vi "Parse GSA Sentence.vi"(8 "error in (no error)":errorcluster, 11 "GSA sentence":string) -> (0 "error out":errorcluster, 3 "GSA data":T1 {"type of fix"."mode" items=["", "No Fix", "2D Fix", "3D Fix"]; "selection of fix"."selection of 2D or 3D fix" items=["Automatic", "Manual"]})   [LabVIEW 2011, in "u-blox 5 Series.lvlib"]
doc: "Returns data contained in an NMEA sentence. You must manually select the polymorphic instance to use."
uses:
  u-blox 5 Series.lvlib
  typedefs/GSA Data.ctl
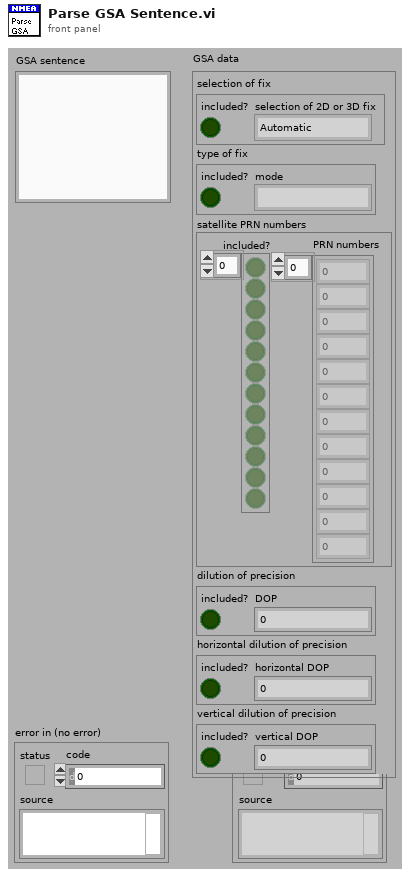
[diagram p1: front panel]
types:
  T1 = typedef "u-blox 5 Series.lvlib/GSA Data.ctl" = cluster{"selection of fix":cluster{"included?":bool, "selection of 2D or 3D fix":u16}, "type of fix":cluster{"included?":bool, "mode":u16}, "satellite PRN numbers":cluster{"included?":bool[], "PRN numbers":i32[]}, "dilution of precision":cluster{"included?":bool, "DOP":dbl}, "horizontal dilution of precision":cluster{"included?":bool, "horizontal DOP":dbl}, "vertical dilution of precision":cluster{"included?":bool, "vertical DOP":dbl}}
  T2 = cluster{"Included?":bool[], "Satellite PRNs":i32[]}
  T3 = cluster{"Valid?":bool, "Selection of 2D or 3D Fix":u16}
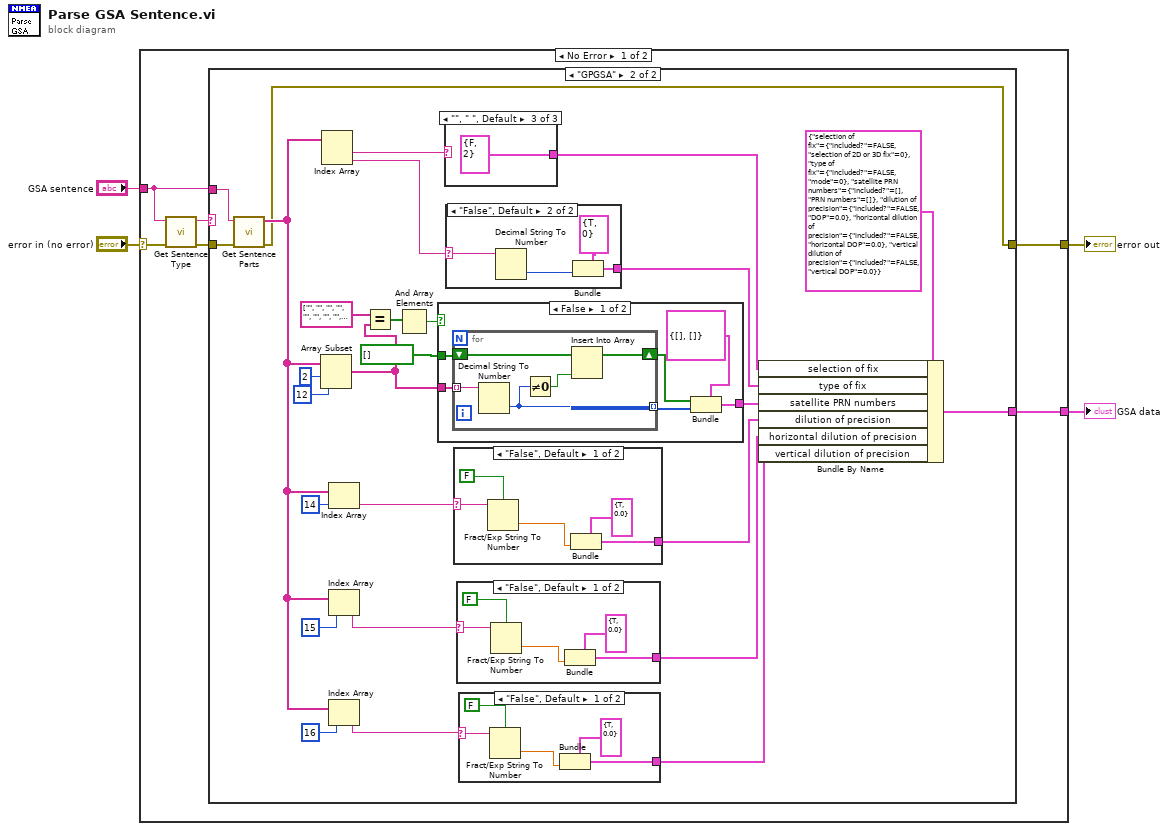
[diagram p0: block diagram]
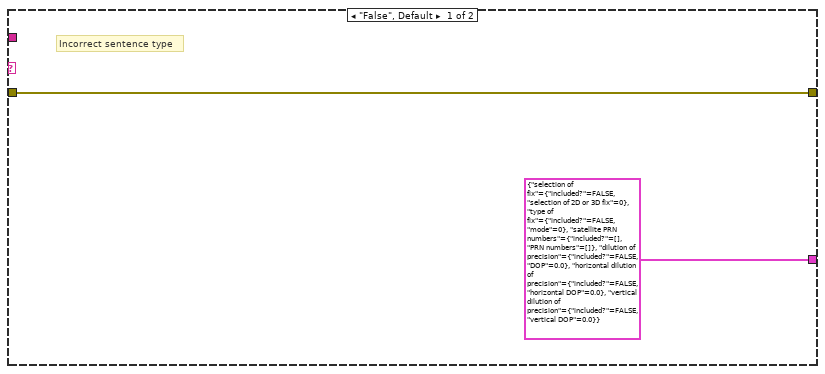
[diagram p2: hidden frame]
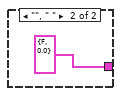
[diagram p3: hidden frame]
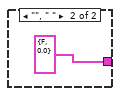
[diagram p4: hidden frame]
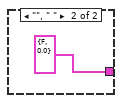
[diagram p5: hidden frame]
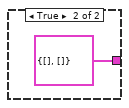
[diagram p6: hidden frame]
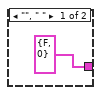
[diagram p7: hidden frame]
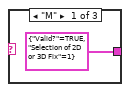
[diagram p8: hidden frame]
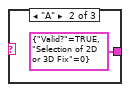
[diagram p9: hidden frame]
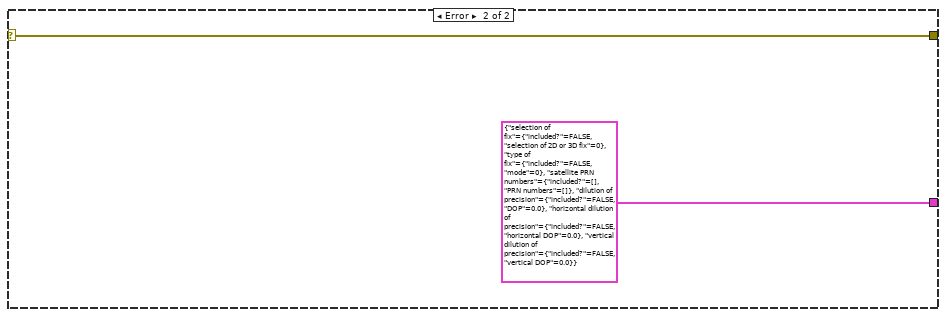
[diagram p10: hidden frame]
diagram:
  n1 = case shown="No Error" "error in (no error)" {
    selector: "error in (no error)" -> [w8 w79]
    tunnel: [w9 w79] -> w2
    tunnel: [w10 T1 {"selection of fix"={"included?"=FALSE, "selection of 2D or 3D fix"=0}, "type of fix"={"included?"=FALSE, "mode"=0}, "satellite PRN numbers"={"included?"=[], "PRN numbers"=[]}, "dilution of precision"={"included?"=FALSE, "DOP"=0.0}, "horizontal dilution of precision"={"included?"=FALSE, "horizontal DOP"=0.0}, "vertical dilution of precision"={"included?"=FALSE, "vertical DOP"=0.0}} ("GSA Data")] -> w1
    tunnel: "GSA sentence" -> [w6 _]
    frame No Error {
      n2 = call "Get Sentence Type.vi"("error in (no error)"=w8, "sentence"=w6) -> ("error out"=w7:errorcluster, "sentence type"=w5:string)  [unwired: 1 in, 7 out]
      n3 = case shown="\"GPGSA\"" w5 {
        tunnel: w6 -> [_ w14]
        tunnel: w7 -> [w11 w39]
        tunnel: [T1 {"selection of fix"={"included?"=FALSE, "selection of 2D or 3D fix"=0}, "type of fix"={"included?"=FALSE, "mode"=0}, "satellite PRN numbers"={"included?"=[], "PRN numbers"=[]}, "dilution of precision"={"included?"=FALSE, "DOP"=0.0}, "horizontal dilution of precision"={"included?"=FALSE, "horizontal DOP"=0.0}, "vertical dilution of precision"={"included?"=FALSE, "vertical DOP"=0.0}} ("GSA Data") w18] -> w10
        tunnel: [w11 w13] -> w9
        frame "False", Default {
          # "Incorrect sentence type"
        }
        frame "GPGSA" {
          n4 = call "Get Sentence Parts.vi"("error in (no error)"=w39, "sentence"=w14) -> ("error out"=w13:errorcluster, "sentence data"=w15:string[])  [unwired: 1 in, 7 out]
          n5 = Array Subset(array=w15, index=2, length=12) -> (w30:string[])
          n6 = Index Array(array=w15) -> (element #1=w38:string, element #2=w34:string)  [unwired: 2 in]
          n7 = Index Array(array=w15, index=14) -> (element=w25:string)
          n8 = Index Array(array=w15, index=15) -> (element=w23:string)
          n9 = Index Array(array=w15, index=16) -> (element=w21:string)
          n10 = Equal?(x=string[] ["", "", "", "", "", "", "", "", "", "", "", ""], y=w30) -> (x = y?=w28:bool[])
          n11 = And Array Elements(Boolean array=w28) -> (logical AND=w27:bool)
          n12 = case shown="False" w27 {
            tunnel: w30 -> [w63 _]
            tunnel: [w60 T2 {"Included?"=[], "Satellite PRNs"=[]} ("Satellite PRNs")] -> w17
            tunnel: bool[] [] ("Included?") -> [w59 _]
            frame False {
              n13 = for {
                tunnel: [w64] -> w62 mode=indexing
                tunnel: w63 -> [w68] mode=indexing
                shift-right: [w66] -> w58
                shift-left: w59 -> [w67]
                n14 = Decimal String To Number(string=w68) -> (number=w64:i32)  [unwired: 3 out]
                n15 = Not Equal To 0?(x=w64) -> (x != 0?=w65:bool)
                n16 = Insert Into Array(array=w67, new element=w65) -> (w66:bool[])  [unwired: 1 in]
              }
              n17 = Bundle(cluster=T2 {"Included?"=[], "Satellite PRNs"=[]} ("Satellite PRNs"), "Included?"=w58, "Satellite PRNs"=w62) -> (w60:T2)
            }
            frame True {
            }
          }
          n18 = case shown="\"\", \" \", Default" w38 {
            tunnel: [T3 {"Valid?"=TRUE, "Selection of 2D or 3D Fix"=1} ("Selection of Fix") T3 {"Valid?"=TRUE, "Selection of 2D or 3D Fix"=0} ("Selection of Fix") T3 {"Valid?"=FALSE, "Selection of 2D or 3D Fix"=2} ("Selection of Fix")] -> w33
            frame "M" {
            }
            frame "A" {
            }
            frame "", " ", Default {
            }
          }
          n19 = case shown="\"False\", Default" w34 {
            selector: w34 -> [_ w74]
            tunnel: [cluster{"Valid?":bool, "Type of Fix":u16} {"Valid?"=FALSE, "Type of Fix"=0} ("Type of Fix") w71] -> w26
            frame "", " " {
            }
            frame "False", Default {
              n20 = Decimal String To Number(string=w74) -> (number=w72:i32)  [unwired: 3 out]
              n21 = Bundle(cluster=cluster{"Valid?":bool, "Type of Fix":u16} {"Valid?"=TRUE, "Type of Fix"=0} ("Type of Fix"), "Type of Fix"=w72) -> (w71:cluster{"Valid?":bool, "Type of Fix":u16})  [unwired: 1 out]
            }
          }
          n22 = case shown="\"False\", Default" w25 {
            selector: w25 -> [w56 _]
            tunnel: [w53 cluster{"Valid?":bool, "DOP":dbl} {"Valid?"=FALSE, "DOP"=0.0} ("Dilution of Precision")] -> w24
            frame "False", Default {
              n23 = Fract/Exp String To Number(use system decimal point (T)=FALSE, string=w56) -> (number=w54:dbl)  [unwired: 3 out]
              n24 = Bundle(cluster=cluster{"Valid?":bool, "DOP":dbl} {"Valid?"=TRUE, "DOP"=0.0} ("Dilution of Precision"), "DOP"=w54) -> (w53:cluster{"Valid?":bool, "DOP":dbl})  [unwired: 1 out]
            }
            frame "", " " {
            }
          }
          n25 = case shown="\"False\", Default" w23 {
            selector: w23 -> [w50 _]
            tunnel: [w47 cluster{"Valid?":bool, "DOP":dbl} {"Valid?"=FALSE, "DOP"=0.0} ("Dilution of Precision")] -> w22
            frame "False", Default {
              n26 = Fract/Exp String To Number(use system decimal point (T)=FALSE, string=w50) -> (number=w48:dbl)  [unwired: 3 out]
              n27 = Bundle(cluster=cluster{"Valid?":bool, "DOP":dbl} {"Valid?"=TRUE, "DOP"=0.0} ("Dilution of Precision"), "DOP"=w48) -> (w47:cluster{"Valid?":bool, "DOP":dbl})  [unwired: 1 out]
            }
            frame "", " " {
            }
          }
          n28 = case shown="\"False\", Default" w21 {
            selector: w21 -> [w44 _]
            tunnel: [w41 cluster{"Valid?":bool, "DOP":dbl} {"Valid?"=FALSE, "DOP"=0.0} ("Dilution of Precision")] -> w20
            frame "False", Default {
              n29 = Fract/Exp String To Number(use system decimal point (T)=FALSE, string=w44) -> (number=w42:dbl)  [unwired: 3 out]
              n30 = Bundle(cluster=cluster{"Valid?":bool, "DOP":dbl} {"Valid?"=TRUE, "DOP"=0.0} ("Dilution of Precision"), "DOP"=w42) -> (w41:cluster{"Valid?":bool, "DOP":dbl})  [unwired: 1 out]
            }
            frame "", " " {
            }
          }
          n31 = Bundle By Name(cluster=T1 {"selection of fix"={"included?"=FALSE, "selection of 2D or 3D fix"=0}, "type of fix"={"included?"=FALSE, "mode"=0}, "satellite PRN numbers"={"included?"=[], "PRN numbers"=[]}, "dilution of precision"={"included?"=FALSE, "DOP"=0.0}, "horizontal dilution of precision"={"included?"=FALSE, "horizontal DOP"=0.0}, "vertical dilution of precision"={"included?"=FALSE, "vertical DOP"=0.0}} ("GSA Data"), "selection of fix"=w33, "type of fix"=w26, "satellite PRN numbers"=w17, "dilution of precision"=w24, "horizontal dilution of precision"=w22, "vertical dilution of precision"=w20) -> (w18:T1)
        }
      }
    }
    frame Error {
    }
  }
  "error out" <- w2
  "GSA data" <- w1
